vi "Find Nested LV XML.vi"(8 "error in (no error)":errorcluster, 11 "Projext Path":path) -> (0 "error out":errorcluster, 2 "lvlibs":path[](array[path]), 3 "lvprojs":path[](array[path]))   [LabVIEW 2020, in "Test Finder.lvclass"]
uses:
  Test Finder.lvclass
  Test Finder.lvclass/Test Finder.ctl
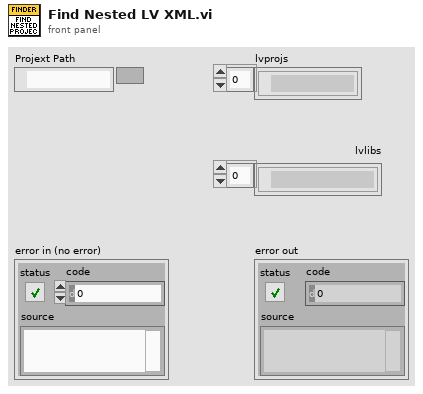
[diagram p1: front panel]
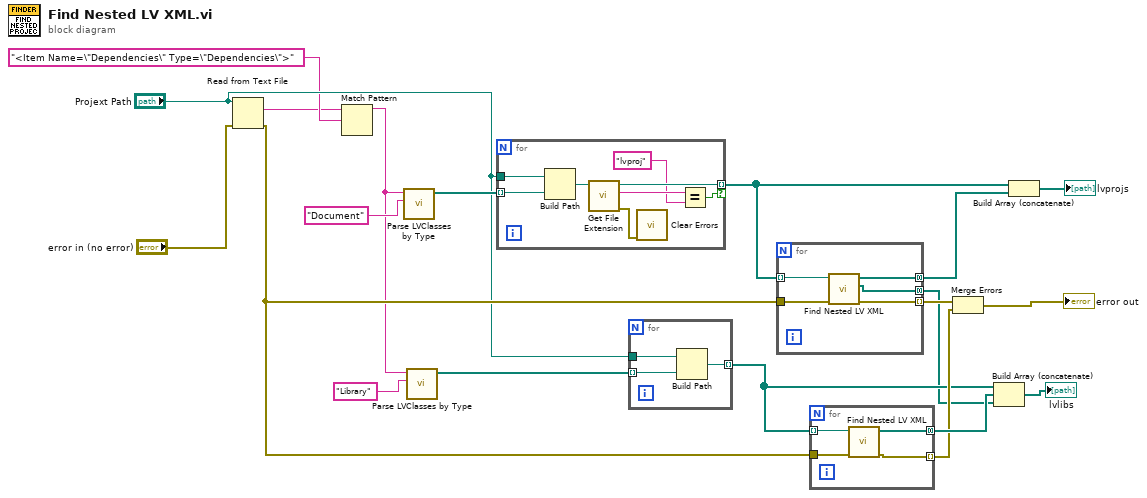
[diagram p0: block diagram]
diagram:
  n1 = Read from Text File(file (use dialog)="Projext Path", error in="error in (no error)") -> (text=w2:string, error out=w19:errorcluster)  [unwired: 2 in, 2 out]
  n2 = Match Pattern(string=w2, regular expression="<Item Name=\"Dependencies\" Type=\"Dependencies\">") -> (before substring=w1:string)  [unwired: 1 in, 3 out]
  n3 = call "Parse LVClasses by Type.vi"("Type"="Document", "Input"=w1) -> ("Relative Paths"=w17:path[])  [unwired: 9 in]
  n4 = call "Parse LVClasses by Type.vi"("Type"="Library", "Input"=w1) -> ("Relative Paths"=w7:path[])  [unwired: 9 in]
  n5 = for {
    tunnel: "Projext Path" -> [w28]
    tunnel: w17 -> [w27] mode=indexing
    tunnel: [w25] -> w16 mode=indexing if=w21
    n6 = Build Path(base path=w28, name or relative path=w27) -> (appended path=w26:path)
    n7 = call <vilib>:"Get File Extension.vi"("file"=w26) -> ("error out"=w22:errorcluster, "lowercase file extension"=w24:string, "dup file"=w25:path)  [unwired: 6 in, 2 out]
    n8 = call <vilib>:"Clear Errors.vi"("error in (no error)"=w22) -> ()  [unwired: 5 in, 2 out]
    n9 = Equal?(x=w24, y="lvproj") -> (x = y?=w21:bool)
  }
  n10 = for {
    tunnel: "Projext Path" -> [w31]
    tunnel: w7 -> [w30] mode=indexing
    tunnel: [w29] -> w6 mode=indexing
    n11 = Build Path(base path=w31, name or relative path=w30) -> (appended path=w29:path)
  }
  n12 = for {
    tunnel: w16 -> [w36] mode=indexing
    tunnel: [w35] -> w14 mode=concatenating
    tunnel: w19 -> [w34]
    tunnel: [w33] -> w13 mode=indexing
    tunnel: [w32] -> w5 mode=concatenating
    n13 = call "Find Nested LV XML.vi"("error in (no error)"=w34, "Projext Path"=w36) -> ("error out"=w33:errorcluster, "lvlibs"=w32:path[], "lvprojs"=w35:path[])  [unwired: 7 in]
  }
  n14 = for {
    tunnel: w6 -> [w40] mode=indexing
    tunnel: [w39] -> w9 mode=concatenating
    tunnel: w19 -> [w38]
    tunnel: [w37] -> w8 mode=indexing
    n15 = call "Find Nested LV XML.vi"("error in (no error)"=w38, "Projext Path"=w40) -> ("error out"=w37:errorcluster, "lvprojs"=w39:path[])  [unwired: 7 in, 1 out]
  }
  n16 = Merge Errors(w13, w8) -> (→"error out":errorcluster)
  n17 = Build Array (concatenate)(w6, w9, w5) -> (→"lvlibs":path[])
  n18 = Build Array (concatenate)(w16, w14) -> (→"lvprojs":path[])
